vi "AR Amplifier control.vi"() -> ()   [LabVIEW 2020]
panel:
  in  "init":bool
  out "Status":string
  in  "Read state":bool
  in  "Stop Button":bool
  in  "Reset":bool
  in  "Power":bool
  in  "Adjust":i32(knob)=100 scale=0.0..100.0
  in  "VISA resource name":refnum<visa-resource-name>
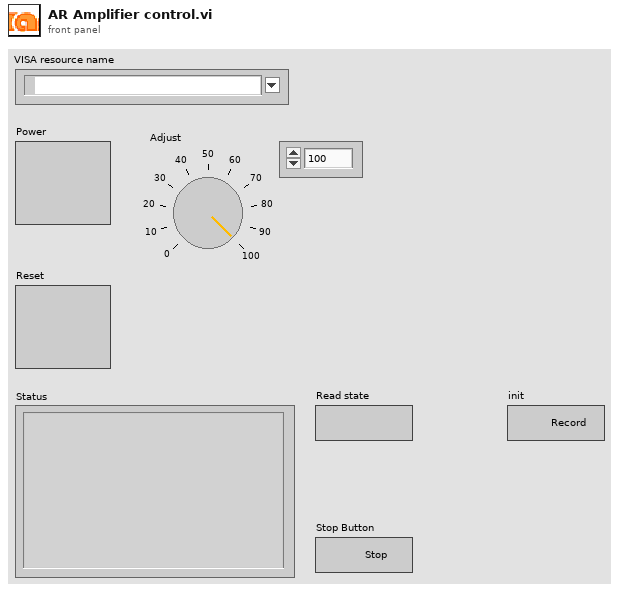
[diagram p1: front panel]
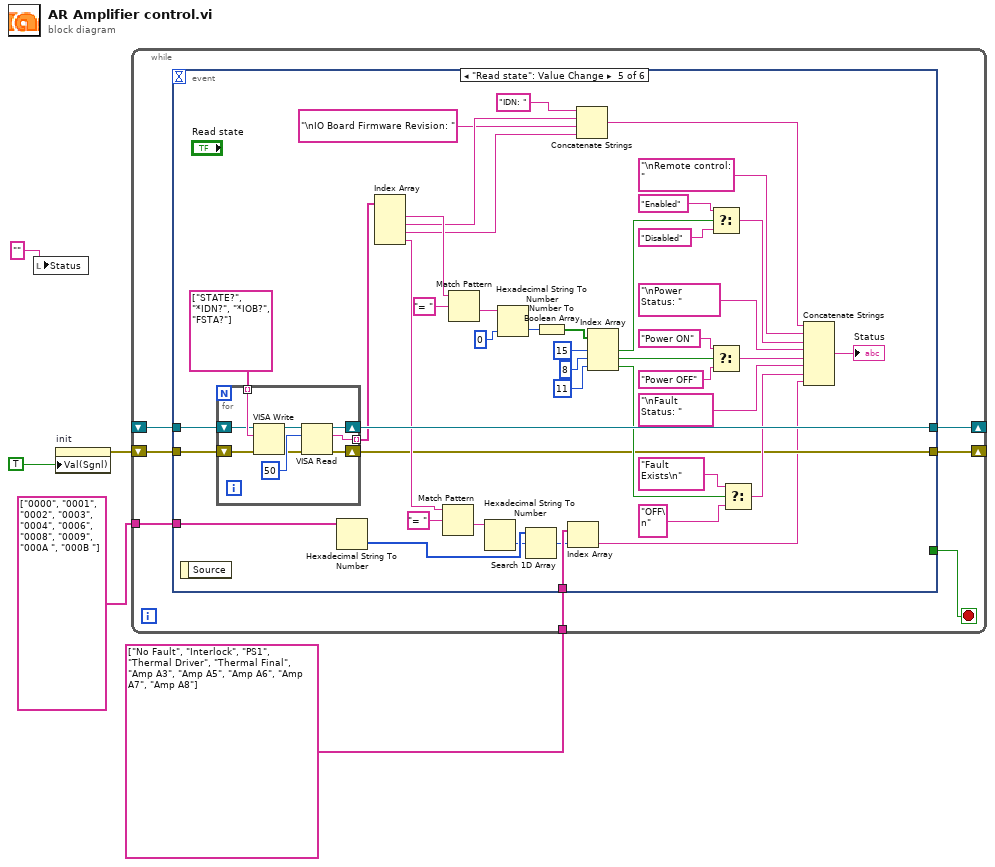
[diagram p0: block diagram]
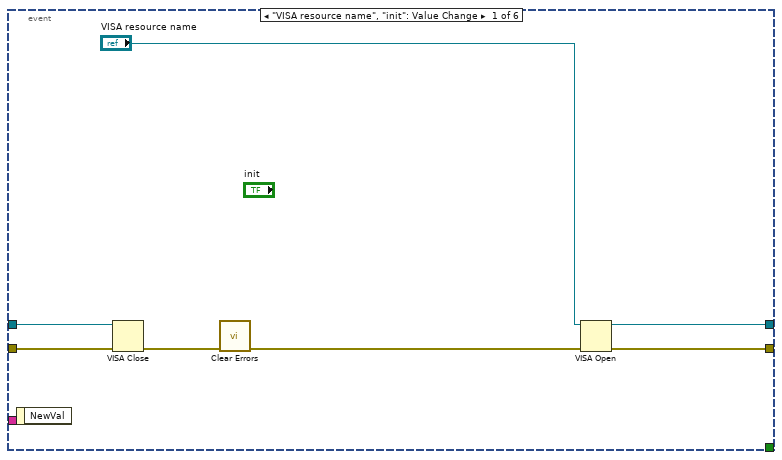
[diagram p2: hidden frame]
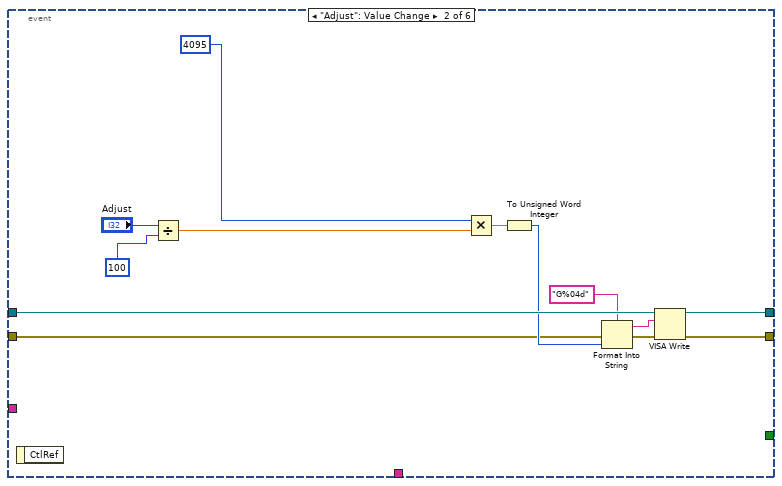
[diagram p3: hidden frame]
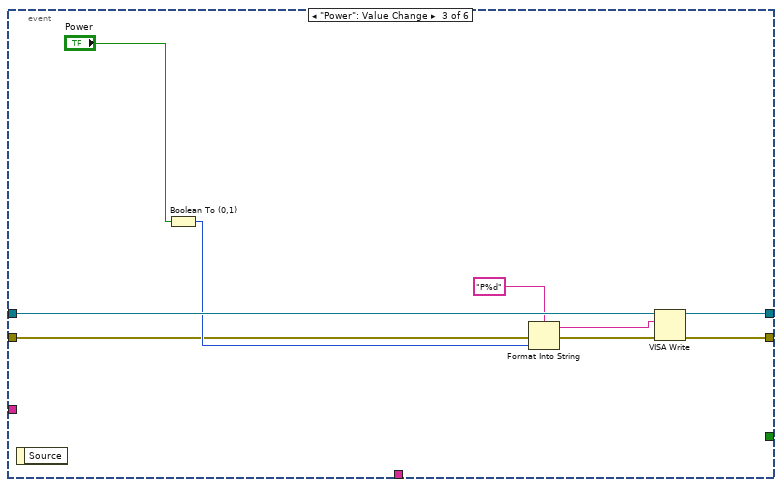
[diagram p4: hidden frame]
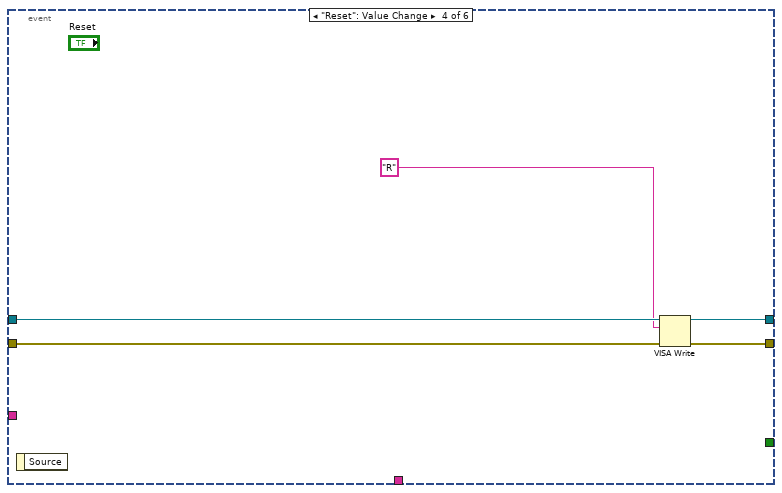
[diagram p5: hidden frame]
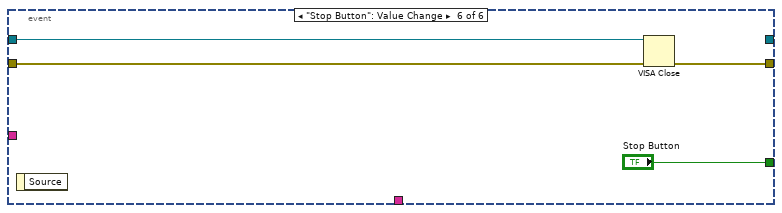
[diagram p6: hidden frame]
diagram:
  n1 = local write "Status"("" ("Status")) -> ()
  n2 = property on="init" class="Bool (strict)"("Val(Sgnl)"=TRUE) -> (error out=w1:errorcluster)  [unwired: 2 in, 1 out]
  n3 = while {
    shift-right: [w12] -> _
    shift-left: _ -> [w11]
    tunnel: string[] ["0000", "0001", "0002", "0003", "0004", "0006", "0008", "0009", "000A ", "000B "] ("Array") -> [w8]
    tunnel: string[] ["No Fault", "Interlock", "PS1", "Thermal Driver", "Thermal Final", "Amp A3", "Amp A5", "Amp A6", "Amp A7", "Amp A8"] ("Array 2") -> [w7]
    shift-right: [w6] -> _
    shift-left: w1 -> [w9]
    stop <- w10 stop-if-true
    n4 = event shown="[4] \"Read state\": Value Change" {
      selector: _ -> [_ _ _ _ _ _]
      dyn-events: _ -> [_ _ _ _ _ _]
      timeout: _ -> [_ _ _ _ _ _]
      tunnel: [w17 w26 w40 w46 w89 _] -> w12
      tunnel: w11 -> [w16 w27 w41 w45 w90 w103]
      tunnel: [_ _ _ _ _ "Stop Button"] -> w10
      tunnel: w9 -> [w14 w21 w34 w42 w88 w101]
      tunnel: w8 -> [_ _ _ _ w51 _]
      tunnel: w7 -> [_ _ _ _ w56 _]
      tunnel: [w13 w22 w33 w43 w53 w102] -> w6
      event "VISA resource name", "init": Value Change {
        n5 = event-data() -> ()  [unwired: 1 in, 1 out]
        n6 = VISA Close(VISA resource name=w16, error in (no error)=w14) -> (error out=w19:errorcluster)
        n7 = call <vilib>:"Clear Errors.vi"("error in (no error)"=w19) -> ("error out"=w18:errorcluster)  [unwired: 5 in, 1 out]
        n8 = VISA Open(error in (no error)=w18, VISA resource name="VISA resource name") -> (VISA resource name=w17:refnum<visa-resource-name>, error out=w13:errorcluster)  [unwired: 3 in]
      }
      event "Adjust": Value Change {
        n9 = event-data() -> ()  [unwired: 1 in, 1 out]
        n10 = Divide(x="Adjust", y=100) -> (x/y=w29:dbl)
        n11 = Multiply(x=4095, y=w29) -> (x*y=w28:dbl)
        n12 = To Unsigned Word Integer(number=w28) -> (unsigned 16bit integer=w24:u16)
        n13 = Format Into String(format string="G%04d", error in=w21, w24) -> (resulting string=w23:string, error out=w20:errorcluster)  [unwired: 1 in]
        n14 = VISA Write(VISA resource name=w27, write buffer=w23, error in (no error)=w20) -> (VISA resource name out=w26:refnum<visa-resource-name>, error out=w22:errorcluster)  [unwired: 1 out]
      }
      event "Power": Value Change {
        n15 = event-data() -> ()  [unwired: 1 in, 1 out]
        n16 = Boolean To (0,1)(Boolean="Power") -> (0, 1=w37:i16)
        n17 = Format Into String(format string="P%d", error in=w34, w37) -> (resulting string=w36:string, error out=w35:errorcluster)  [unwired: 1 in]
        n18 = VISA Write(VISA resource name=w41, write buffer=w36, error in (no error)=w35) -> (VISA resource name out=w40:refnum<visa-resource-name>, error out=w33:errorcluster)  [unwired: 1 out]
      }
      event "Reset": Value Change {
        n19 = event-data() -> ()  [unwired: 1 in, 1 out]
        n20 = VISA Write(VISA resource name=w45, write buffer="R", error in (no error)=w42) -> (VISA resource name out=w46:refnum<visa-resource-name>, error out=w43:errorcluster)  [unwired: 1 out]
      }
      event "Read state": Value Change {
        n21 = event-data() -> ()  [unwired: 1 in, 1 out]
        n22 = for {
          tunnel: string[] ["STATE?", "*IDN?", "*IOB?", "FSTA?"] -> [w100] mode=indexing
          shift-right: [w97] -> w89
          shift-left: w90 -> [w99]
          tunnel: [w96] -> w63 mode=indexing
          shift-right: [w92] -> w53
          shift-left: w88 -> [w93]
          n23 = VISA Write(VISA resource name=w99, write buffer=w100, error in (no error)=w93) -> (VISA resource name out=w98:refnum<visa-resource-name>, error out=w94:errorcluster)  [unwired: 1 out]
          n24 = VISA Read(VISA resource name=w98, byte count=u32 50, error in (no error)=w94) -> (VISA resource name out=w97:refnum<visa-resource-name>, read buffer=w96:string, error out=w92:errorcluster)  [unwired: 1 out]
        }
        n25 = Hexadecimal String To Number(string=w51) -> (number=w50:u32[])  [unwired: 2 in, 1 out]
        n26 = Index Array(array=w63) -> (element #1=w87:string, element #2=w61:string, element #3=w59:string, element #4=w57:string)  [unwired: 4 in]
        n27 = Match Pattern(string=w57, regular expression="= ") -> (after substring=w49:string)  [unwired: 1 in, 3 out]
        n28 = Match Pattern(string=w87, regular expression="= ") -> (after substring=w85:string)  [unwired: 1 in, 3 out]
        n29 = Hexadecimal String To Number(string=w49) -> (number=w48:u32)  [unwired: 2 in, 1 out]
        n30 = Hexadecimal String To Number(string=w85, default (0uL)=u16 0) -> (number=w84:u16)  [unwired: 1 in, 1 out]
        n31 = Search 1D Array(1D array=w50, element=w48) -> (index of element=w55:i32)  [unwired: 1 in]
        n32 = Number To Boolean Array(number=w84) -> (Boolean array=w47:bool[])
        n33 = Index Array(array=w56, index=w55) -> (element=w52:string)
        n34 = Concatenate Strings("IDN: ", w61, "\nIO Board Firmware Revision: ", w59) -> (w54:string)
        n35 = Index Array(array=w47, index #1=15 ("index"), index #2=8 ("index"), index #3=11 ("index")) -> (element #1=w78:bool, element #2=w77:bool, element #3=w79:bool)
        n36 = Select(t="Enabled", s=w78, f="Disabled") -> (s? t:f=w75:string)
        n37 = Select(t="Power ON", s=w77, f="Power OFF") -> (s? t:f=w67:string)
        n38 = Select(t="Fault Exists\n", s=w79, f="OFF\n") -> (s? t:f=w65:string)
        n39 = Concatenate Strings(w54, "\nRemote control: ", w75, "\nPower Status: ", w67, "\nFault Status: ", w65, w52) -> (→"Status":string)
      }
      event "Stop Button": Value Change {
        n40 = event-data() -> ()  [unwired: 1 in, 1 out]
        n41 = VISA Close(VISA resource name=w103, error in (no error)=w101) -> (error out=w102:errorcluster)
      }
    }
  }
